vi "Filter_CW.vi"() -> (5 "Plug in titles":string[](array[string]), 7 "Plug in values":string[](array[string]))   [LabVIEW 2011]
uses:
  Globals/Plug_in_data_global.vi
  Globals/Meas_global.vi
  <vilib>/Analysis/3filter.llb/Butterworth Filter (DBL).vi
  <vilib>/Analysis/NI_AALBase.lvlib
panel:
  out "Waveform Graph":dbl[][](graph)
  # "Run this VI to update the channel names"
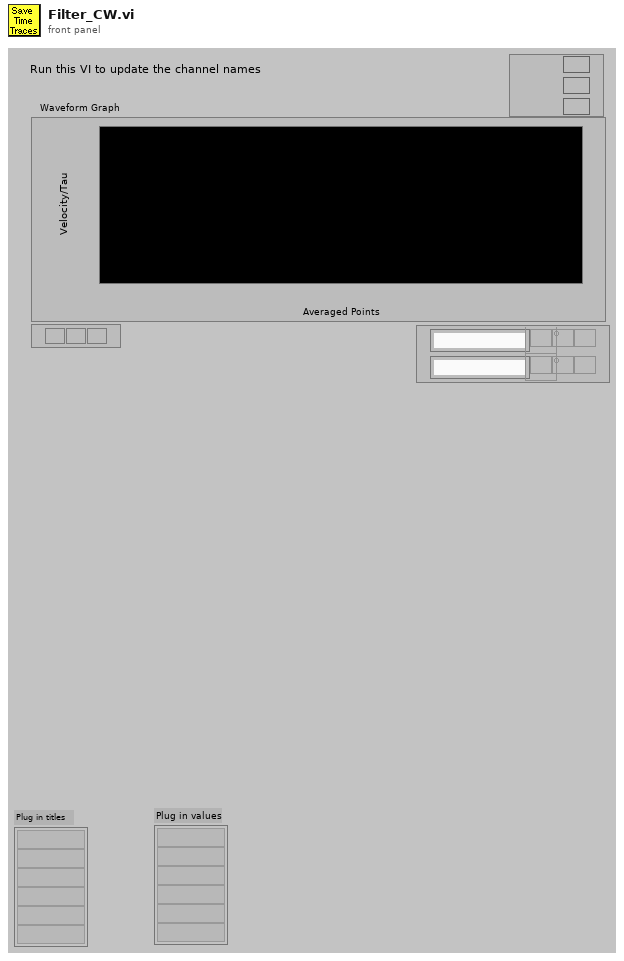
[diagram p1: front panel]
types:
  T1 = enum32{"Lowpass", "Highpass", "Bandpass", "Bandstop"}
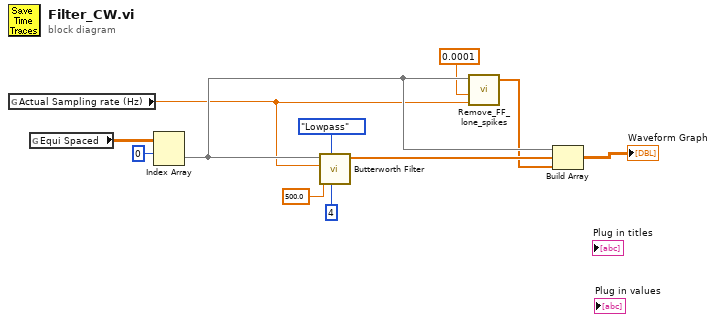
[diagram p0: block diagram]
diagram:
  n1 = global read "Meas_global.vi" "Actual Sampling rate (Hz)"() -> (w2:dbl)
  n2 = global read "Plug_in_data_global.vi" "Equi Spaced"() -> (w11:dbl[][])
  n3 = Index Array(array=w11, index (row)=0) -> (element=w5:dbl[])  [unwired: 1 in]
  n4 = call-poly <vilib>:"Butterworth Filter.vi"("order"=4, "filter type"=T1."Lowpass", "low cutoff freq: fl"=500.0 ("high cutoff freq: fh"), "sampling freq: fs"=w2, "X"=w5) -> ("Filtered X"=w8:dbl[])  [unwired: 2 in, 2 out]
  n5 = call "Remove_FF_lone_spikes.vi"("ADC Frequency Hz"=w2, "Bkgnd variance"=0.0001, "Time Trace"=w5) -> ("Filtered Time Trace"=w1:dbl[])  [unwired: 1 in, 2 out]
  n6 = Build Array(w5, w8, w1) -> (→"Waveform Graph":dbl[][])
